vi "Connect.vi"(8 "error in (no error)":errorcluster, 11 "SimulationMotor in":refnum<class "SimulationMotor.lvclass">) -> (0 "error out":errorcluster, 2 "Is Connected":bool, 3 "SimulationMotor out":refnum<class "SimulationMotor.lvclass">)   [LabVIEW 2016, in "SimulationMotor.lvclass"]
doc: "This VI establishes a connection to the motor drive.\n\n<b>Copyright (C) 2018 Control Software Solutions Limited. All rights reserved. </b>"
uses:
  SimulationMotor.lvclass
panel:
  in  "Is Connected Control":bool
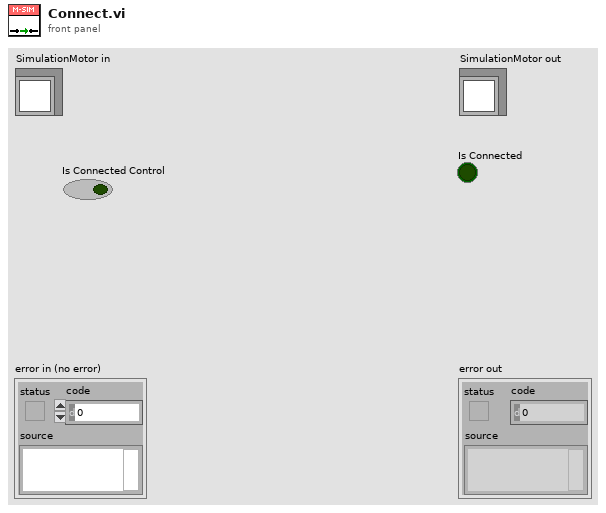
[diagram p1: front panel]
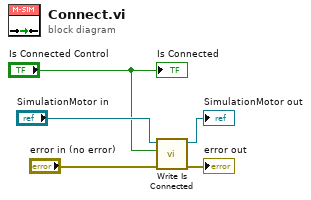
[diagram p0: block diagram]
diagram:
  n1 = call-dynamic "Write Is Connected.vi"("error in (no error)"="error in (no error)", "Is Connected"="Is Connected Control", "MotorDrive in"="SimulationMotor in") -> ("error out"=→"error out":errorcluster, "MotorDrive out"=→"SimulationMotor out":refnum<class "SimulationMotor.lvclass">)  [unwired: 7 in]
  "Is Connected" <- "Is Connected Control"
